vi "Write to block memory.vi"() -> ()   [LabVIEW 2014]
uses:
  <vilib>/rvi/interface/nirviOpenFPGA/nirviOpenFPGA.xnode
  <vilib>/rvi/interface/nirviMethod/nirviMethod.xnode
  <vilib>/rvi/errors/niLvFpgaMergeErrorWithErrorCode.vi
  <vilib>/rvi/interface/nirviCloseFPGA/nirviCloseFPGA.xnode
  Write elements to FIFO and Process on sha.vi
  <vilib>/rvi/interface/nirviReadWriteControl/nirviReadWriteControl.xnode
  NiFpgaLv.dll
  <vilib>/Utility/error.llb/Error Cluster From Error Code.vi
  <vilib>/rvi/interface/Simulation/niFpgaSimulationCallBeginRW.vi
  <vilib>/rvi/errors/niLvFpgaAdjustHostInterfaceError.vi
  <vilib>/rvi/DesktopExecutionNode/DesktopExecutionNode.xnode
  <vilib>/rvi/DesktopExecutionNode/Execution/niFpgaDEN_Execute.vi
  <vilib>/rvi/interface/RandomDataEmulation/nirviRandomDataOpen.vi
  <vilib>/rvi/interface/common/niFpgaCacheSessionInfoDynamic.vi
  <vilib>/FPGAPlugInAG/Dynamic/niLvFpga_StopFifo_Dynamic.vi
  <vilib>/FPGAPlugInAG/Dynamic/niLvFpga_StartFifo_Dynamic.vi
  <vilib>/FPGAPlugInAG/Dynamic/niLvFpga_WriteFifo_Dynamic.vi
  <vilib>/FPGAPlugInAG/Dynamic/niLvFpga_Close_Dynamic.vi
panel:
  out "output array":u8[](array[numeric])
  out "FIFO Output":u8[](array[numeric])
  out "Digest":u8[](array[numeric])
  out "Empty Elements Remaining":u32
  in  "error in":errorcluster
  in  "Send Data?":bool
  out "End of File?":bool
  out "error out":errorcluster
  out "text":string
  in  "stop":bool
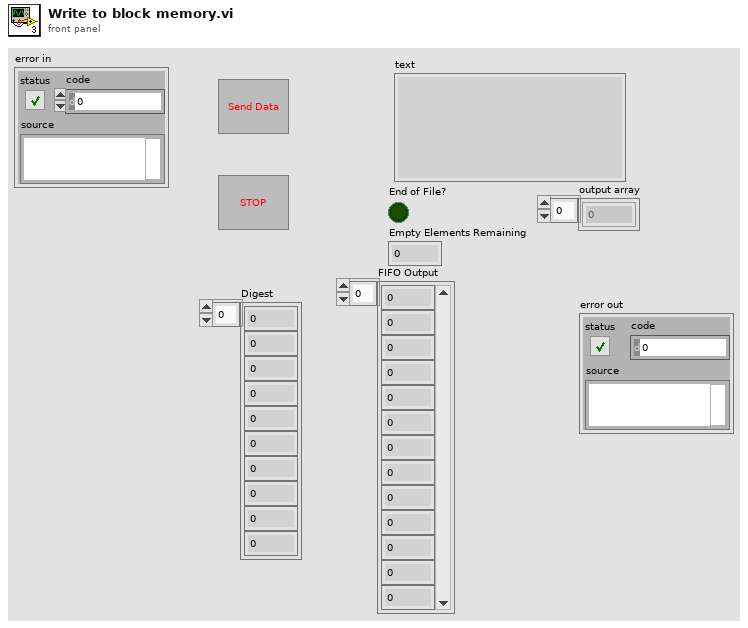
[diagram p1: front panel]
types:
  T1 = enum16{"open", "replace", "create", "open or create", "replace or create", "replace or create with confirmation"}
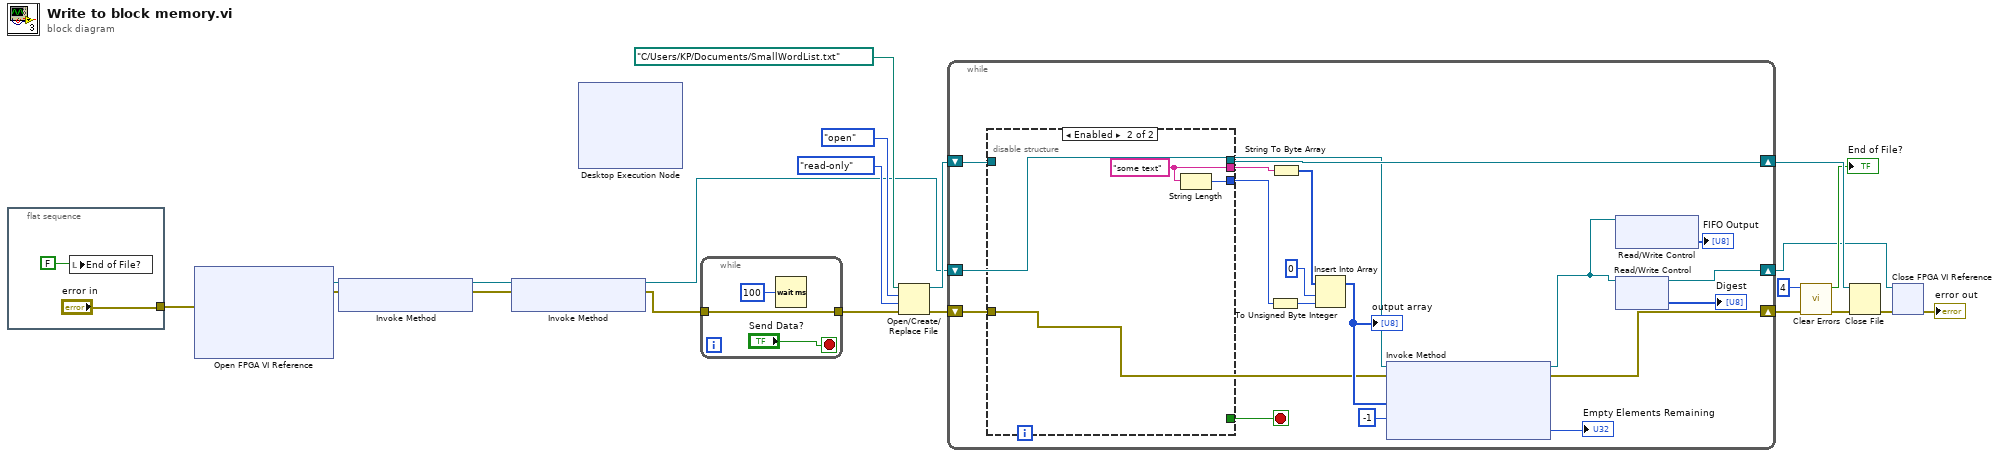
[diagram p0: block diagram]
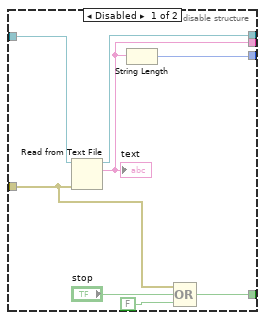
[diagram p2: hidden frame]
diagram:
  n1 = flat-sequence {
    tunnel: ["error in"] -> w1
    frame #0 {
      n2 = local write "End of File?"(FALSE) -> ()
    }
  }
  n3 = xnode "Open FPGA VI Reference"("error in"=w1) -> ("FPGA VI Reference Out"=w7:refnum<k20>, "error out"=w4:errorcluster)  [unwired: 1 in]
  n4 = xnode "Invoke Method"("FPGA VI Reference In"=w7, "error in"=w4) -> ("FPGA VI Reference Out"=w6:refnum<k20>, "error out"=w3:errorcluster)
  n5 = xnode "Invoke Method"("FPGA VI Reference In"=w6, "error in"=w3) -> ("FPGA VI Reference Out"=w5:refnum<k20>, "error out"=w2:errorcluster)
  n6 = xnode "Desktop Execution Node"() -> ()  [unwired: 1 in, 1 out]
  n7 = while {
    tunnel: [w24] -> w12
    tunnel: w2 -> [w24]
    stop <- "Send Data?" stop-if-true
    n8 = Wait (ms)(milliseconds to wait=u32 100) -> ()  [unwired: 1 out]
  }
  n9 = Open/Create/Replace File(file path (use dialog)=path "C:/Users/KP/Documents/SmallWordList.txt", error in=w12, operation (0:open)=T1."open", access (0:read/write)=enum16{"read/write", "read-only", "write-only"}."read-only") -> (refnum out=w18:refnum<file>, error out=w13:errorcluster)  [unwired: 2 in, 1 out]
  n10 = while {
    shift-right: [w30] -> w11
    shift-left: w5 -> [w39]
    shift-right: [w33] -> w10
    shift-left: w13 -> [w27]
    shift-right: [w43] -> w17
    shift-left: w18 -> [w44]
    stop <- w42 stop-if-true
    n11 = disable-structure shown="Enabled" {
      disable-tunnel: w44 -> [w52 _]
      disable-tunnel: [w51 _] -> w43
      disable-tunnel: [w49 _] -> w42
      disable-tunnel: [w47 w53] -> w41
      disable-tunnel: [w46 w54] -> w40
      disable-tunnel: w27 -> [w45 _]
      frame Disabled {
        n12 = Read from Text File(file (use dialog)=w52, error in=w45) -> (refnum out=w51:refnum<file>, text=w46:string)  [unwired: 2 in, 2 out]
        "text" <- w46
        n13 = String Length(string=w46) -> (length=w47:i32)
        n14 = Compound Arithmetic op=OR(w45, "stop", FALSE ("y")) -> (w49:bool)
      }
      frame Enabled {
        w54 = "some text"
        n15 = String Length(string=w54) -> (length=w53:i32)
      }
    }
    n16 = To Unsigned Byte Integer(number=w41) -> (unsigned 8bit integer=w37:u8)
    n17 = String To Byte Array(string=w40) -> (unsigned byte array=w35:u8[])
    n18 = Insert Into Array(array=w35, index=0 ("Timeout"), new element=w37) -> (w34:u8[])
    "output array" <- w34
    n19 = xnode "Invoke Method"("FPGA VI Reference In"=w39, "error in"=w27, "Data"=w34, "Timeout (ms)"=-1 ("Timeout")) -> ("FPGA VI Reference Out"=w29:refnum<k20>, "error out"=w33:errorcluster, "Empty Elements Remaining"=→"Empty Elements Remaining":u32)
    n20 = xnode "Read/Write Control"("FPGA VI Reference In"=w29) -> ("FIFO Output"=→"FIFO Output":u8[])  [unwired: 1 in, 2 out]
    n21 = xnode "Read/Write Control"("FPGA VI Reference In"=w29) -> ("FPGA VI Reference Out"=w30:refnum<k20>, "Digest"=→"Digest":u8[])  [unwired: 1 in, 1 out]
  }
  n22 = call <vilib>:"Clear Errors.vi"("error in (no error)"=w10, "specific error code to clear (0: all)"=4) -> ("error out"=w15:errorcluster, "specific error cleared?"=→"End of File?":bool)  [unwired: 4 in]
  n23 = Close File(refnum=w17, error in=w15) -> (error out=w9:errorcluster)  [unwired: 1 out]
  n24 = xnode "Close FPGA VI Reference"("FPGA VI Reference In"=w11, "error in"=w9) -> ("error out"=→"error out":errorcluster)
